vi "Parse OM.vi"(8 "error in (no error)":errorcluster, 11 "OM in":string) -> (0 "error out":errorcluster, 3 "OM out":T1)   [LabVIEW 2018, in "Config_Read_BML.lvclass"]
uses:
  Config_Read_BML.lvclass
  OperationMode.ctl
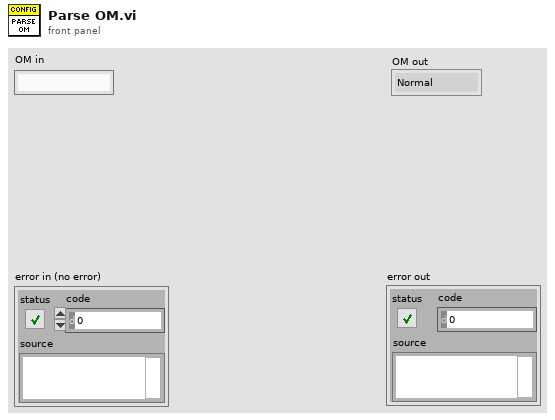
[diagram p1: front panel]
types:
  T1 = typedef "Config_Read_BML.lvclass/OperationMode.ctl" = enum8{"Normal", "ImmeEffect", "InitSlaveID", "LoadData"}
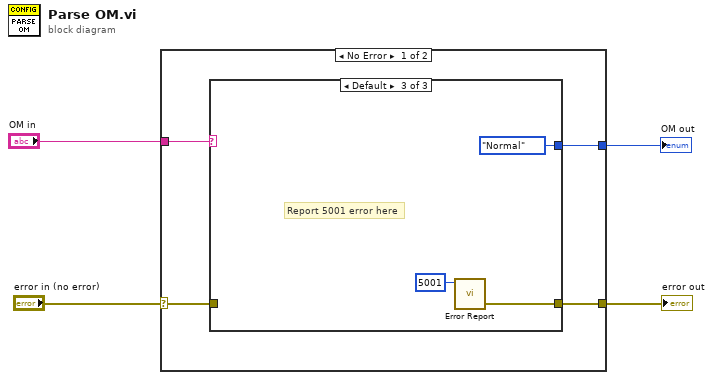
[diagram p0: block diagram]
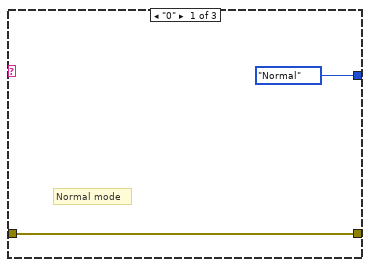
[diagram p2: hidden frame]
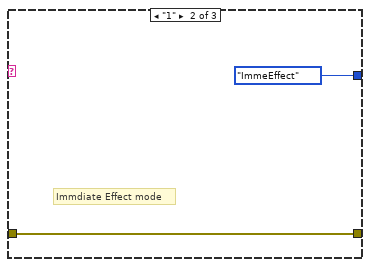
[diagram p3: hidden frame]
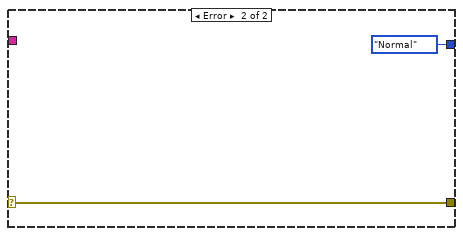
[diagram p4: hidden frame]
diagram:
  n1 = case shown="No Error" "error in (no error)" {
    selector: "error in (no error)" -> [w8 w17]
    tunnel: "OM in" -> [w7 _]
    tunnel: [w6 OperationMode."Normal" ("OM out")] -> w2
    tunnel: [w5 w17] -> w1
    frame No Error {
      n2 = case shown="Default" w7 {
        tunnel: w8 -> [w9 w11 _]
        tunnel: [OperationMode."Normal" ("OM out") OperationMode."ImmeEffect" ("OM out") OperationMode."Normal" ("OM out")] -> w6
        tunnel: [w9 w11 w13] -> w5
        frame "0" {
          # "Normal mode"
        }
        frame "1" {
          # "Immdiate Effect mode"
        }
        frame Default {
          # "Report 5001 error here"
          n3 = call "Error Report.vi"("Error Code"=i16 5001) -> ("error out"=w13:errorcluster)  [unwired: 10 in]
        }
      }
    }
    frame Error {
    }
  }
  "OM out" <- w2
  "error out" <- w1
